vi "Global - Monitoring Variables.vi"() -> ()   [LabVIEW 2013]
panel:
  in  "Send Live Data":bool caption="发送实时数据"
  in  "Live Data Channel":u32 caption="实时数据通道"
  in  "Drive Space":dbl caption="驱动器空间"
  in  "Buffer Backlog":dbl caption="缓冲区积压"
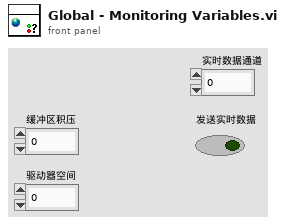
[diagram p1: front panel]
diagram:
